vi "MechanicalActions.vi"() -> ()   [LabVIEW 2015]
panel:
  in  "stop":bool
  in  "Push\nButton 6":bool
  out "LED 6":bool
  out "LED 5":bool
  in  "Push\nButton 5":bool
  in  "Push\nButton 4":bool
  out "LED 4":bool
  out "LED 3":bool
  in  "Push\nButton 3":bool
  in  "Push\nButton 2":bool
  out "LED 2":bool
  out "LED":bool
  in  "Push\nButton":bool
  # "Acciones Mecanicas de Botones"
  # "Serrano Bermúdez Luis Esteban\nFecha de Entrega 23/02/2019"
  # "Desecripcion: Explicación de las acciones mecánicas que tienen los\n                     botones en LabVIEW"
  # "Switch when\nRelased"
  # "Switch when\nPressed"
  # "El resultado de dar click sobre\nel botón se ve reflejado\ninmediatamente y cambia\nhasta que se vuelve a presionar."
  # "El resultado del boton se\nrefleja hasta que es liberado\nel botón, cambia hasta que se\npresiona de nuevo."
  # "Latch when \nPressed"
  # "Switch until\nReleased"
  # "La acción se ve unicamente\nmientras se mantenga\npresionado el botón. Cambia\nal soltarse."
  # "El resultado de dar click sobre\nel botón se ve reflejado\ninmediatamente y cambia\nhasta que LabVIEW lee el dato."
  # "Latch until\nReleased"
  # "Latch when\nReleased"
  # "El resultado del boton se\nrefleja hasta que es liberado\nel botón, cambia hasta que\nLabVIEW lee el dato."
  # "La acción se ve unicamente\nmientras se mantenga\npresionado el botón. Cambia\nhasta que LabVIEW lee el dato."
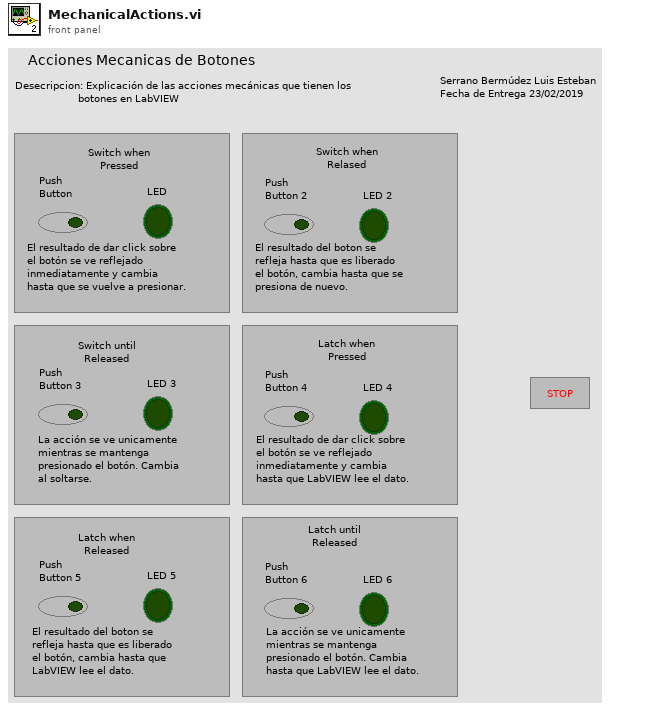
[diagram p1: front panel]
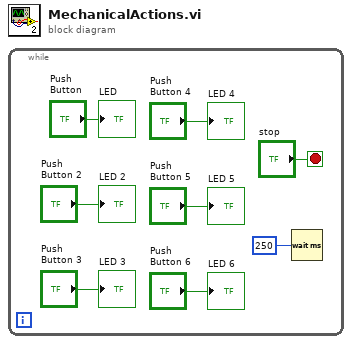
[diagram p0: block diagram]
diagram:
  n1 = while {
    stop <- "stop" stop-if-true
    n2 = Wait (ms)(milliseconds to wait=u32 250) -> ()  [unwired: 1 out]
    "LED" <- "Push\nButton"
    "LED 2" <- "Push\nButton 2"
    "LED 3" <- "Push\nButton 3"
    "LED 4" <- "Push\nButton 4"
    "LED 5" <- "Push\nButton 5"
    "LED 6" <- "Push\nButton 6"
  }
